vi "Sample Cycle.vi"(8 "Error In":errorcluster) -> ()   [LabVIEW 2016]
uses:
  ZI Lockin/ZI Lockin.lvclass
  ZI Lockin/Write Address.vi
  <instrlib>/Zurich Instruments LabOne/Zurich Instruments LabOne.lvlib
panel:
  out "Nodes":string[](array[string])
  out "Array":string[](array[string])
  in  "ZI Address":string
  in  "S":u32
  in  "Stop Button":bool
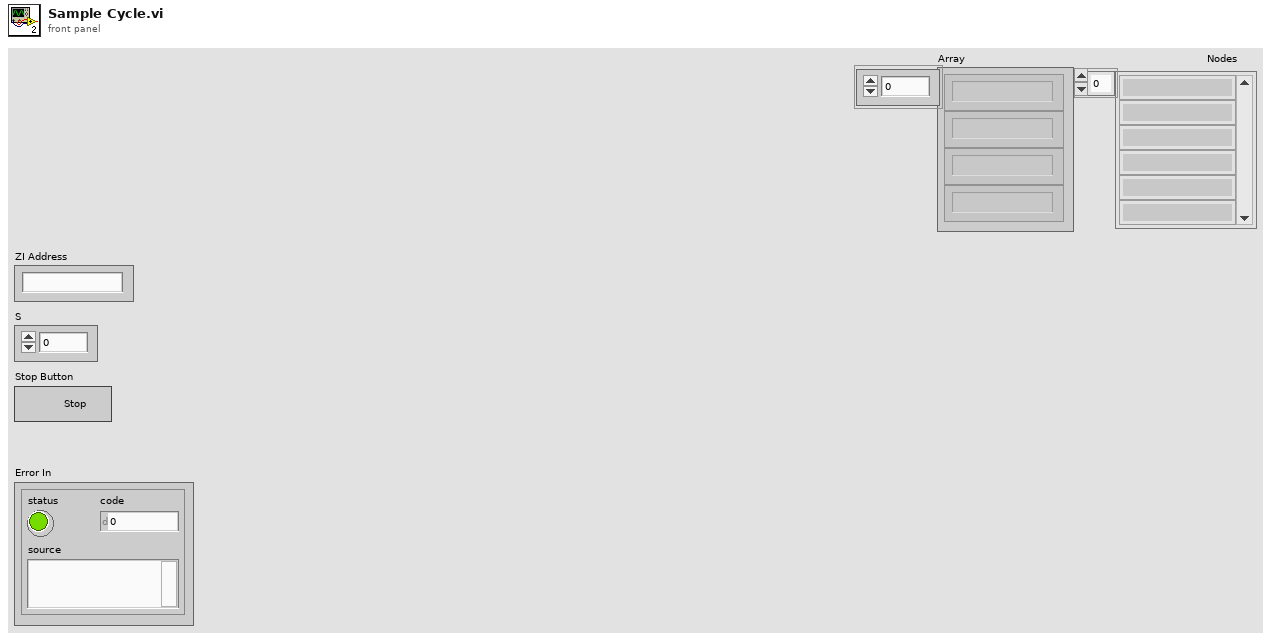
[diagram p1: front panel]
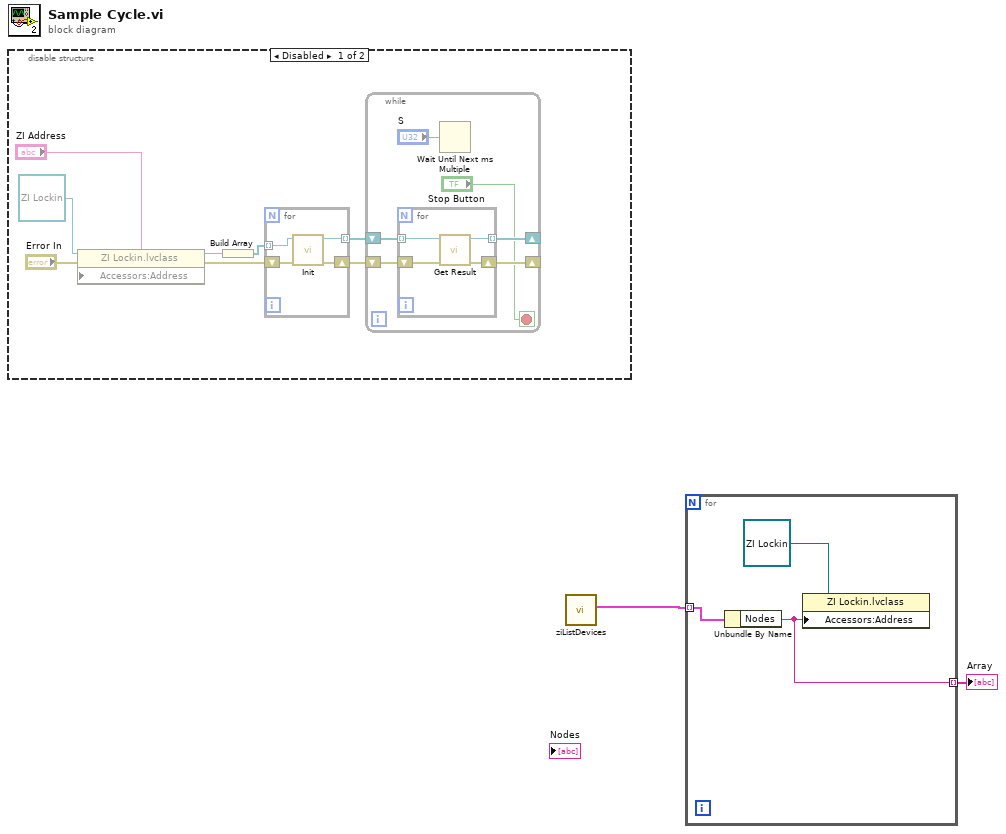
[diagram p0: block diagram]
diagram:
  n1 = disable-structure shown="Disabled" {
    frame Disabled {
      n2 = property class="ZI Lockin.lvclass"(reference=refnum<class "ZI Lockin.lvclass"> refnum ("ZI Lockin.lvclass"), error in="Error In", "Accessors:Address"="ZI Address") -> (reference out=w4:refnum<class "ZI Lockin.lvclass">, error out=w6:errorcluster)
      n3 = Build Array(w4) -> (w9:refnum<class "ZI Lockin.lvclass">[])
      n4 = for {
        tunnel: w9 -> [w24] mode=indexing
        tunnel: [w23] -> w8 mode=indexing
        shift-right: [w21] -> w7
        shift-left: w6 -> [w22]
        n5 = call-dynamic "Init.vi"("error in (no error)"=w22, "Instrument Driver in"=w24) -> ("error out"=w21:errorcluster, "Instrument Driver out"=w23:refnum<class "ZI Lockin.lvclass">)  [unwired: 7 in, 1 out]
      }
      n6 = while {
        shift-right: [w14] -> _
        shift-left: w8 -> [w16]
        shift-right: [w13] -> _
        shift-left: w7 -> [w15]
        stop <- "Stop Button" stop-if-true
        n7 = for {
          tunnel: w16 -> [w20] mode=indexing
          tunnel: [w18] -> w14 mode=indexing
          shift-right: [w17] -> w13
          shift-left: w15 -> [w19]
          n8 = call-dynamic "Get Result.vi"("error in (no error)"=w19, "ZI Lockin in"=w20) -> ("error out"=w17:errorcluster, "ZI Lockin out"=w18:refnum<class "ZI Lockin.lvclass">)  [unwired: 7 in, 1 out]
        }
        n9 = Wait Until Next ms Multiple(millisecond multiple="S") -> ()  [unwired: 1 out]
      }
    }
    frame Enabled {
    }
  }
  n10 = call <instrlib>:"ziListDevices.vi"() -> ("Devices"=w2:cluster{"Nodes":string, i32}[])  [unwired: 5 in, 2 out]
  n11 = for {
    tunnel: w2 -> [w26] mode=indexing
    tunnel: [w25] -> w1 mode=indexing
    n12 = Unbundle By Name(w26) -> ("Nodes"=w25:string)
    n13 = property class="ZI Lockin.lvclass"(reference=refnum<class "ZI Lockin.lvclass"> refnum ("ZI Lockin.lvclass"), "Accessors:Address"=w25) -> ()  [unwired: 1 in, 2 out]
  }
  "Array" <- w1
